vi "Bézier curve.vi"(1 "Spacing":dbl, 2 "Parameters":cluster{"X":dbl, "Y":dbl}[](array[cluster])) -> (0 "Coordinate Array":cluster{"X":dbl, "Y":dbl}[](array[cluster]))   [LabVIEW 2011]
doc: "This VI uses the equation for a Bézier curve to create a set of coordinates."
panel:
  out "XY Graph":cluster{dbl[], dbl[]}[](graph)
  # "Test the Bézier curves"
  # "Formula:    B(t)  =  (1-t)^3 * P0 + 3 * (1-t)^2 * t * P1 + 3 * (1-t) * t^2 * P2 + t^3 * P3"
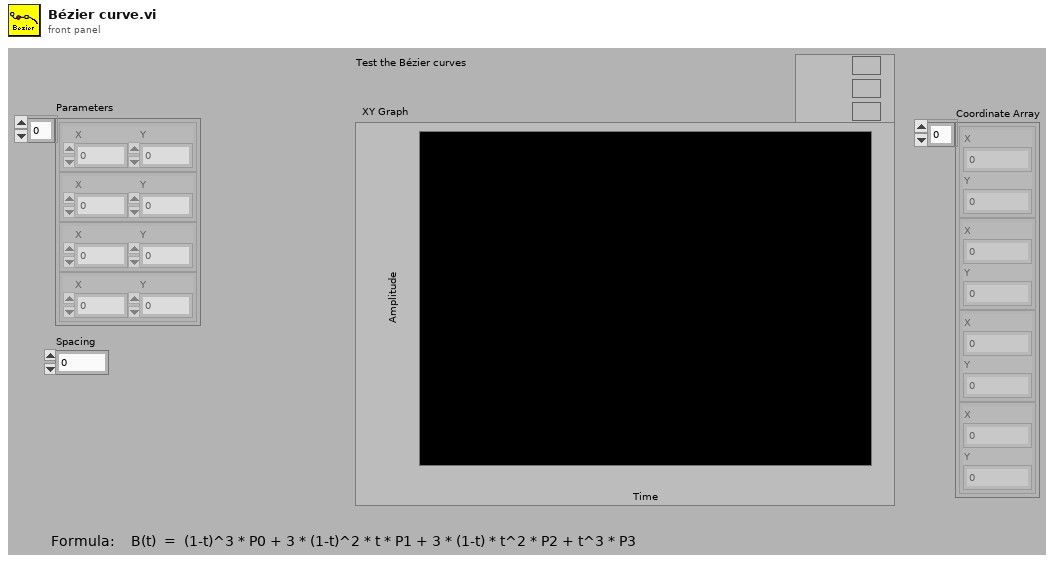
[diagram p1: front panel]
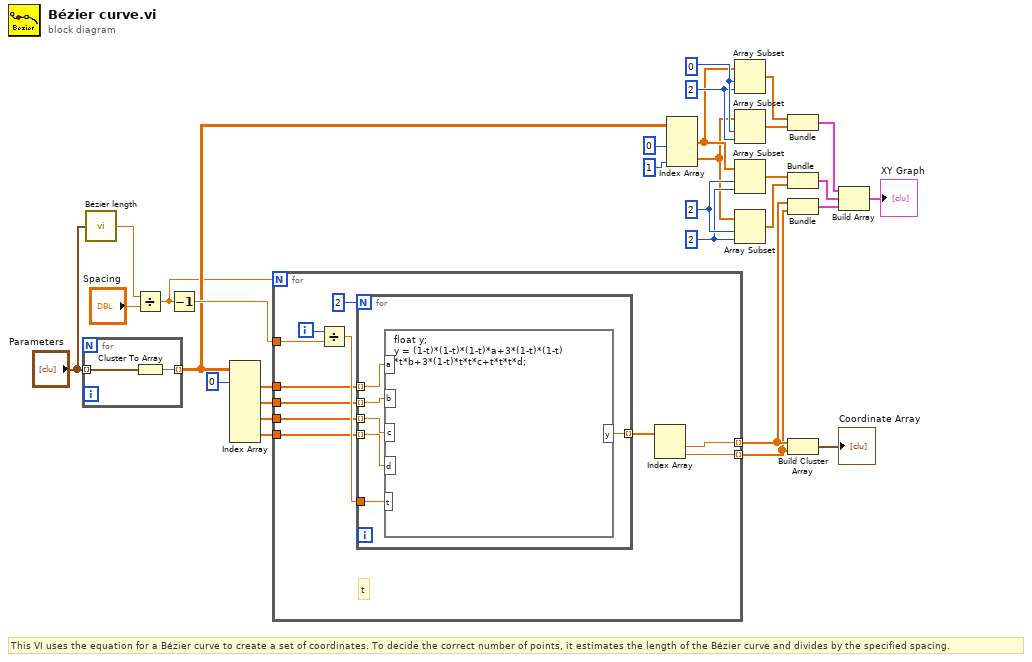
[diagram p0: block diagram]
diagram:
  w25 = 2 ("length")
  w26 = 2 ("index")
  w27 = 2 ("length")
  w28 = 0 ("index")
  # "This VI uses the equation for a Bézier curve to create a set of coordinates. To decide the correct number of points, it estimates the length of the Bézier curve and divides by the specified spacing."
  n1 = for {
    tunnel: "Parameters" -> [w32] mode=indexing
    tunnel: [w31] -> w5 mode=indexing
    n2 = Cluster To Array(cluster=w32) -> (array=w31:dbl[])
  }
  n3 = call "Bézier length.vi"("Parameters"="Parameters") -> ("Length"=w3:dbl)
  n4 = Divide(x=w3, y="Spacing") -> (x/y=w2:dbl)
  n5 = Decrement(x=w2) -> (x-1=w15:dbl)
  n6 = Index Array(array=w5, index (row) #1=0 ("index (row)")) -> (element #1=w13:dbl[], element #2=w12:dbl[], element #3=w11:dbl[], element #4=w10:dbl[])  [unwired: 7 in]
  n7 = for {
    N: w2 -> [_]
    tunnel: w13 -> [w40]
    tunnel: w15 -> [w42]
    tunnel: w12 -> [w39]
    tunnel: w11 -> [w38]
    tunnel: w10 -> [w37]
    tunnel: [w35] -> w8 mode=indexing
    tunnel: [w34] -> w7 mode=indexing
    i -> [w43]
    # "t"
    n8 = Divide(x=w43, y=w42) -> (x/y=w41:dbl)
    n9 = for {
      N: 2 -> [_]
      tunnel: w41 -> [w49]
      tunnel: w40 -> [w48] mode=indexing
      tunnel: w39 -> [w47] mode=indexing
      tunnel: w38 -> [w46] mode=indexing
      tunnel: w37 -> [w45] mode=indexing
      tunnel: [w44] -> w36 mode=indexing
      n10 = formula code="float y;\ny = (1-t)*(1-t)*(1-t)*a+3*(1-t)*(1-t)\n*t*b+3*(1-t)*t*t*c+t*t*t*d;"("t"=w49, "a"=w48, "b"=w47, "c"=w46, "d"=w45) -> ("y"=w44:dbl)
    }
    n11 = Index Array(array=w36) -> (element #1=w35:dbl, element #2=w34:dbl)  [unwired: 2 in]
  }
  n12 = Index Array(array=w5, index (col) #1=0 ("disabled index (col)"), index (col) #2=1 ("index (col)")) -> (element #1=w24:dbl[], element #2=w9:dbl[])  [unwired: 2 in]
  n13 = Array Subset(array=w24, index=w28, length=w27) -> (w20:dbl[])
  n14 = Array Subset(array=w9, index=w28, length=w27) -> (w19:dbl[])
  n15 = Array Subset(array=w24, index=w26, length=w25) -> (w18:dbl[])
  n16 = Array Subset(array=w9, index=w26, length=w25) -> (w17:dbl[])
  n17 = Bundle(w20, w19) -> (w23:cluster{dbl[], dbl[]})  [unwired: 1 in]
  n18 = Bundle(w18, w17) -> (w22:cluster{dbl[], dbl[]})  [unwired: 1 in]
  n19 = Bundle(w8, w7) -> (w16:cluster{dbl[], dbl[]})  [unwired: 1 in]
  n20 = Build Cluster Array(w8, w7) -> (→"Coordinate Array":cluster{dbl, dbl}[])
  n21 = Build Array(w23, w22, w16) -> (→"XY Graph":cluster{dbl[], dbl[]}[])
